vi "俄罗斯方块-消除满行.vi"(11 "输入数组":u32[][](array[colorbox])) -> (0 "行数":u32, 1 "分数":u32, 3 "输出数组":u32[][](array[colorbox]))   [LabVIEW 2016]
panel:
  out "布尔":bool=TRUE
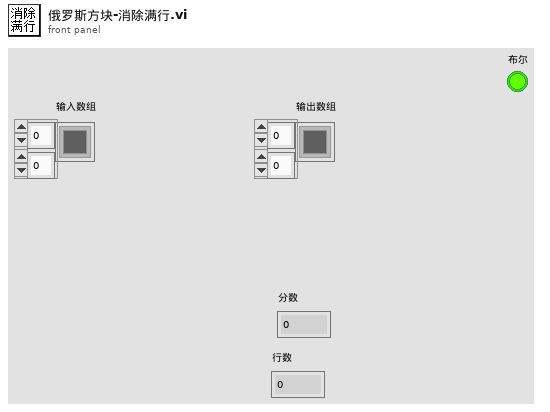
[diagram p1: front panel]
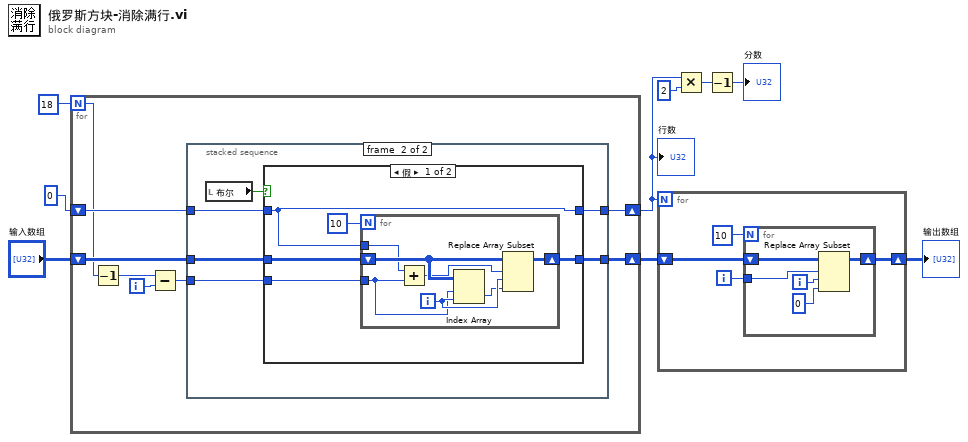
[diagram p0: block diagram]
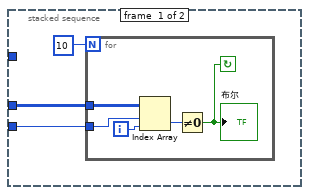
[diagram p2: hidden frame]
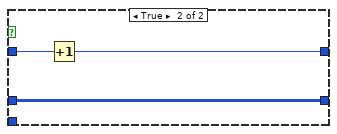
[diagram p3: hidden frame]
diagram:
  n1 = for {
    N: 18 -> [w11]
    shift-right: [w12] -> w3
    shift-left: "输入数组" -> [w17]
    shift-right: [w14] -> w1
    shift-left: u32 0 ("t") -> [w13]
    i -> [w15]
    n2 = Decrement(x=w11) -> (x-1=w10:i32)
    n3 = Subtract(x=w10, y=w15) -> (x-y=w16:i32)
    n4 = stacked-sequence {
      tunnel: w17 -> [w20 w29]
      tunnel: w16 -> [w18 w28]
      tunnel: w13 -> [_ w31]
      tunnel: [_ w30] -> w14
      tunnel: [_ w27] -> w12
      frame #0 {
        n5 = for {
          N: 10 -> [_]
          tunnel: w18 -> [w23]
          tunnel: w20 -> [w24]
          i -> [w21]
          stop <- w25 continue-if-true
          n6 = Index Array(array=w24, index (row)=w23, index (col)=w21) -> (element=w22:u32)
          n7 = Not Equal To 0?(x=w22) -> (x != 0?=w25:bool)
          "布尔" <- w25
        }
      }
      frame #1 {
        n8 = local read "布尔"() -> (w26:bool)
        n9 = case shown="假" w26 {
          tunnel: w31 -> [w32 w46]
          tunnel: [w32 w45] -> w30
          tunnel: w29 -> [w33 w44]
          tunnel: w28 -> [w35 _]
          tunnel: [w34 w44] -> w27
          frame False {
            n10 = for {
              N: 10 -> [_]
              tunnel: w35 -> [w38]
              shift-right: [w43] -> w34
              shift-left: w33 -> [w42]
              tunnel: w32 -> [w37]
              i -> [w41]
              n11 = Add(x=w37, y=w38) -> (x+y=w40:u32)
              n12 = Index Array(array=w42, index (row)=w38, index (col)=w41) -> (element=w39:u32)
              n13 = Replace Array Subset(array=w42, new element=w39, index (row)=w40, index (col)=w41) -> (w43:u32[][])
            }
          }
          frame True {
            n14 = Increment(x=w46) -> (x+1=w45:u32)
          }
        }
      }
    }
  }
  "行数" <- w1
  n15 = for {
    N: w1 -> [_]
    shift-right: [w49] -> w2
    shift-left: w3 -> [w50]
    i -> [w47]
    n16 = for {
      N: 10 -> [_]
      shift-right: [w54] -> w49
      shift-left: w50 -> [w55]
      tunnel: w47 -> [w53]
      i -> [w52]
      n17 = Replace Array Subset(array=w55, new element=u32 0 ("新元素/子数组"), index (row)=w53, index (col)=w52) -> (w54:u32[][])
    }
  }
  "输出数组" <- w2
  n18 = Multiply(x=w1, y=u32 2) -> (x*y=w5:u32)
  n19 = Decrement(x=w5) -> (x-1=→"分数":u32)
